vi "Constant - File Version String.vi"() -> (0 "File Version String (to search for this in output of version.dll:GetFileVersionInfoA)":string)   [LabVIEW 2023, in "Error Manager.lvlib"]
doc: "<add documentation here>"
uses:
  Error Manager.lvlib
panel:
  out "number of replacements":i32
  out "File Version String (Codes Display)":string
  # "Development\ncontrols/indicators useful for development and testing, but which are not outputs of the VI"
  # "Input\nInputs to the VI"
  # "Output\nOutputs of the VI"
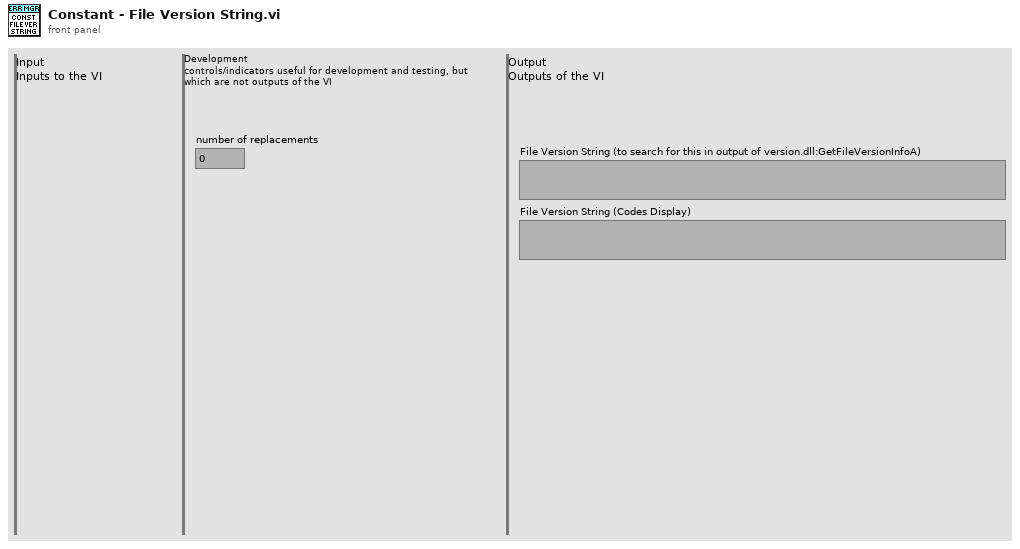
[diagram p1: front panel]
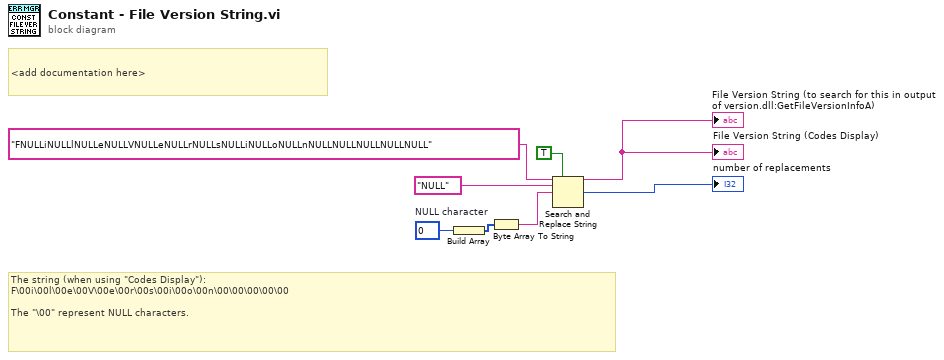
[diagram p0: block diagram]
diagram:
  w6 = u8 0  # NULL character
  # "The string (when using \"Codes Display\"):\nF\\00i\\00l\\00e\\00V\\00e\\00r\\00s\\00i\\00o\\00n\\00\\00\\00\\00\\00\n\nThe \"\\00\" represent NULL characters."
  # "<add documentation here>"
  n1 = Build Array(w6) -> (w5:u8[])
  n2 = Byte Array To String(unsigned byte array=w5) -> (string=w4:string)
  n3 = Search and Replace String(replace all?=TRUE ("replace all? (F)"), input string="FNULLiNULLlNULLeNULLVNULLeNULLrNULLsNULLiNULLoNULLnNULLNULLNULLNULLNULL" ("string"), search string="NULL", replace string=w4) -> (result string=→"File Version String (to search for this in output of version.dll:GetFileVersionInfoA)" →"File Version String (Codes Display)":string, number of replacements=→"number of replacements":i32)  [unwired: 4 in, 2 out]
